vi "Motor write log.vi"(4 "prefix":string, 5 "version":string, 6 "current priority":string, 7 "enabled priority":string, 8 "error in (no error)":errorcluster, 9 "resp array":string[](array[string]), 10 "send array":string[](array[string]), 11 "Motor in":refnum<class "Motor.lvclass">) -> (0 "error out":errorcluster, 1 "error":bool, 2 "logged text":string, 3 "Motor out":refnum<class "Motor.lvclass">)   [LabVIEW 2018, in "Motor.lvclass"]
uses:
  Motor.lvclass
  Motor.lvclass/Motor.ctl
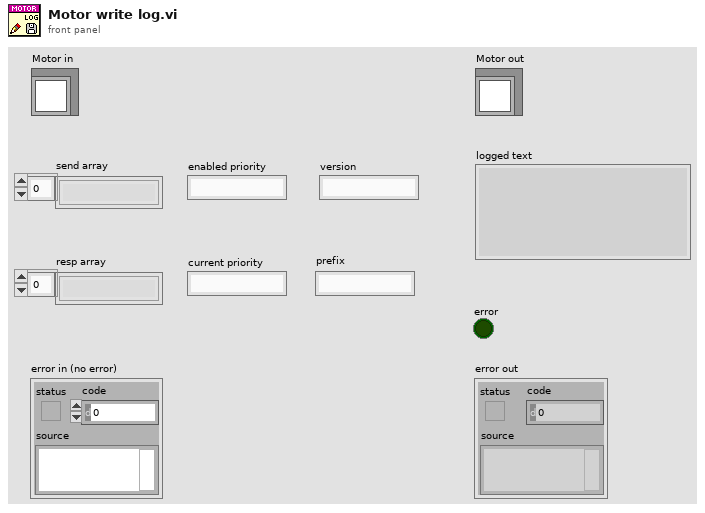
[diagram p1: front panel]
types:
  T1 = enum16{"open", "replace", "create", "open or create", "replace or create", "replace or create with confirmation"}
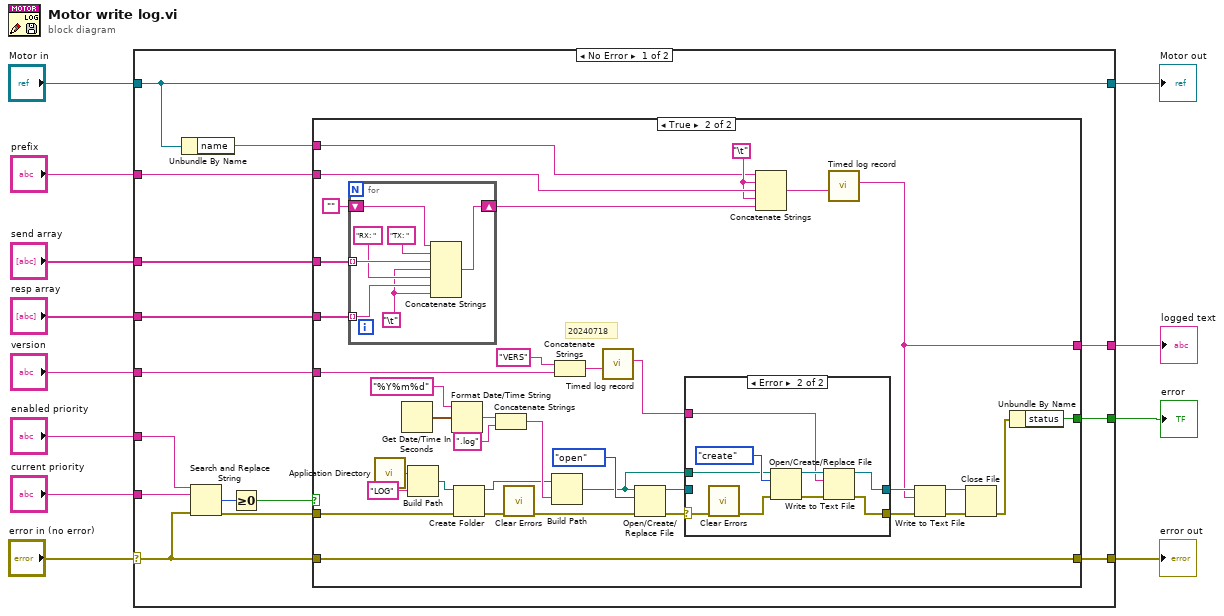
[diagram p0: block diagram]
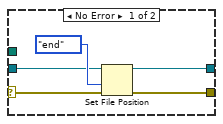
[diagram p3: hidden frame]
diagram:
  n1 = case shown="No Error" "error in (no error)" {
    selector: "error in (no error)" -> [w16 w86]
    tunnel: [w27 w87] -> w10
    tunnel: "Motor in" -> [w27 w87]
    tunnel: "prefix" -> [w26 _]
    tunnel: "send array" -> [w25 _]
    tunnel: "resp array" -> [w24 _]
    tunnel: "enabled priority" -> [w20 _]
    tunnel: "current priority" -> [w19 _]
    tunnel: "version" -> [w18 _]
    tunnel: [w15 w86] -> w3
    tunnel: [w14 _] -> w2
    tunnel: [w13 _] -> w1
    frame No Error {
      n2 = Unbundle By Name(w27) -> ("name"=w17:string)
      n3 = Search and Replace String(input string=w20, search string=w19, error in=w16) -> (number of replacements=w23:i32, error out=w22:errorcluster)  [unwired: 5 in, 2 out]
      n4 = Greater Or Equal To 0?(x=w23) -> (x >= 0?=w21:bool)
      n5 = case shown="True" w21 {
        tunnel: [_ w64] -> w14
        tunnel: w24 -> [_ w63]
        tunnel: w25 -> [_ w62]
        tunnel: [_ w32] -> w13
        tunnel: w26 -> [_ w44]
        tunnel: w22 -> [_ w60]
        tunnel: w18 -> [_ w36]
        tunnel: w17 -> [_ w35]
        tunnel: w16 -> [w28 w34]
        tunnel: [w28 w34] -> w15
        frame False {
        }
        frame True {
          w43 = "\t"
          # "20240718"
          n6 = for {
            tunnel: w63 -> [w83] mode=indexing
            tunnel: w62 -> [w85] mode=indexing
            shift-right: [w80] -> w42
            shift-left: "" -> [w81]
            w79 = "\t"
            n7 = Concatenate Strings(w81, "TX: ", w85, w79, "RX: ", w83, w79) -> (w80:string)
          }
          n8 = call <vilib>:"Application Directory.vi"() -> ("Application Directory"=w59:path)
          n9 = Get Date/Time In Seconds() -> (seconds since 1Jan1904=w57:timestamp)
          n10 = Build Path(base path=w59, name or relative path="LOG") -> (appended path=w49:path)
          n11 = Format Date/Time String(time format string (%c)="%Y%m%d", seconds (now)=w57) -> (date/time string=w55:string)  [unwired: 1 in]
          n12 = Create Folder(path (use dialog)=w49, error in=w60) -> (created path=w46:path, error out=w48:errorcluster)  [unwired: 1 in, 1 out]
          n13 = Concatenate Strings(w55, ".log" ("string")) -> (w54:string)
          n14 = call <vilib>:"Clear Errors.vi"("error in (no error)"=w48) -> ("error out"=w47:errorcluster)  [unwired: 5 in, 1 out]
          n15 = Build Path(base path=w46, name or relative path=w54) -> (appended path=w37:path)
          n16 = Concatenate Strings("VERS" ("string"), w36) -> (w30:string)
          n17 = call "Timed log record .vi"("log input"=w30) -> ("log register"=w29:string)  [unwired: 9 in, 1 out]
          n18 = Open/Create/Replace File(file path (use dialog)=w37, error in=w47, operation (0:open)=T1."open") -> (refnum out=w40:refnum<file>, error out=w41:errorcluster)  [unwired: 3 in, 1 out]
          n19 = case shown="Error" w41 {
            selector: w41 -> [w68 w78]
            tunnel: w40 -> [w67 _]
            tunnel: [w66 w71] -> w39
            tunnel: [w65 w72] -> w38
            tunnel: w37 -> [_ w76]
            tunnel: w29 -> [_ w70]
            frame No Error {
              n20 = Set File Position(refnum=w67, from (0:start)=enum16{"start", "end", "current"}."end", error in=w68) -> (refnum out=w66:refnum<file>, error out=w65:errorcluster)  [unwired: 1 in]
            }
            frame Error {
              n21 = call <vilib>:"Clear Errors.vi"("error in (no error)"=w78) -> ("error out"=w75:errorcluster)  [unwired: 5 in, 1 out]
              n22 = Open/Create/Replace File(file path (use dialog)=w76, error in=w75, operation (0:open)=T1."create") -> (refnum out=w73:refnum<file>, error out=w74:errorcluster)  [unwired: 3 in, 1 out]
              n23 = Write to Text File(file (use dialog)=w73, text=w70, error in=w74) -> (refnum out=w71:refnum<file>, error out=w72:errorcluster)  [unwired: 1 in, 1 out]
            }
          }
          n24 = Concatenate Strings(w35, w43, w44, w43, w42) -> (w33:string)
          n25 = call "Timed log record .vi"("log input"=w33) -> ("log register"=w32:string)  [unwired: 9 in, 1 out]
          n26 = Write to Text File(file (use dialog)=w39, text=w32, error in=w38) -> (refnum out=w52:refnum<file>, error out=w51:errorcluster)  [unwired: 1 in, 1 out]
          n27 = Close File(refnum=w52, error in=w51) -> (error out=w50:errorcluster)  [unwired: 1 out]
          n28 = Unbundle By Name(w50) -> ("status"=w64:bool)
        }
      }
    }
    frame Error {
    }
  }
  "error out" <- w3
  "Motor out" <- w10
  "error" <- w2
  "logged text" <- w1
